vi "RT_Write_DMARS_String.vi"(8 "error in (no error)":errorcluster, 9 "String":string, 11 "FPGA VI Reference Out":refnum<k20>) -> (0 "error out":errorcluster, 3 "FPGA VI Reference Out 2":refnum<k20>)   [LabVIEW 2011]
uses:
  <vilib>/Utility/error.llb/Error Cluster From Error Code.vi
  <vilib>/rvi/errors/niLvFpgaAdjustHostInterfaceError.vi
  <vilib>/RVI Host/nirviSupport.llb/nirviErrorClusterFromErrorCode.vi
  <vilib>/rvi/interface/nirviReadWriteControl/nirviReadWriteControl.xnode
  <vilib>/rvi/interface/nirviMethod/nirviMethod.xnode
  <vilib>/rvi/errors/niLvFpgaMergeErrorWithErrorCode.vi
  <vilib>/FPGAPlugInAG/Dynamic/niLvFpga_WriteFifo_Dynamic.vi
  NiFpgaLv.dll
  <vilib>/rvi/interface/Simulation/niFpgaSimulationCallBeginRW.vi
  <vilib>/rvi/interface/nirviMethod/StockFPGA_InlinedMethodWaitForSingleIRQ.vi
  <vilib>/FPGAPlugInAG/Dynamic/niLvFpga_WaitOnIrq_Dynamic.vi
  <vilib>/FPGAPlugInAG/Dynamic/niLvFpga_AcknowledgeIrq_Dynamic.vi
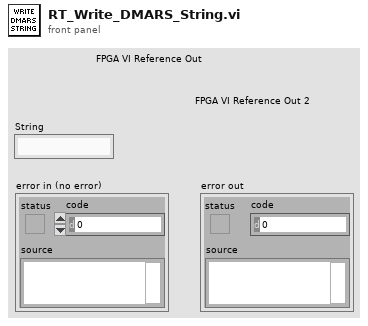
[diagram p1: front panel]
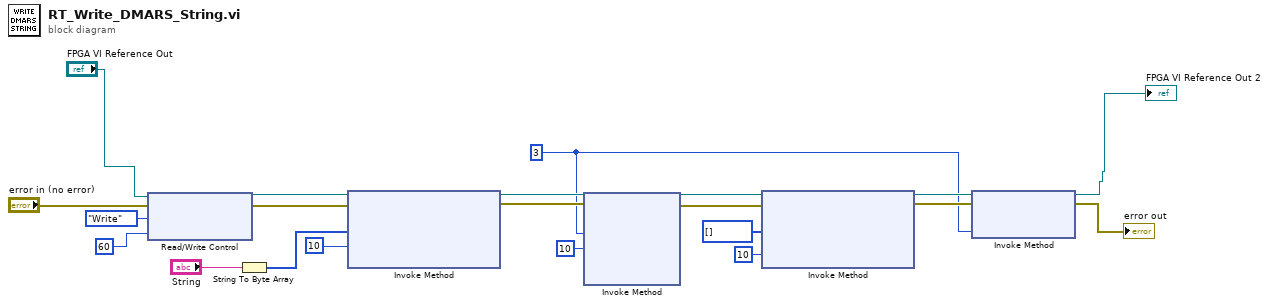
[diagram p0: block diagram]
diagram:
  w6 = 3 ("IRQ Number(s)")
  n1 = xnode "Read/Write Control"("FPGA VI Reference In"="FPGA VI Reference Out", "error in"="error in (no error)", "Op_Write P3"=enum16{"Stand_by", "Write"}."Write" ("Op_Write"), "Bytes-to-Write P3"=60 ("Bytes-to-Read")) -> ("FPGA VI Reference Out"=w10:refnum<k20>, "error out"=w11:errorcluster)
  n2 = String To Byte Array(string="String") -> (unsigned byte array=w20:u8[])
  n3 = xnode "Invoke Method"("FPGA VI Reference In"=w10, "error in"=w11, "Data"=w20, "Timeout (ms)"=10) -> ("FPGA VI Reference Out"=w12:refnum<k20>, "error out"=w13:errorcluster)  [unwired: 1 out]
  n4 = xnode "Invoke Method"("FPGA VI Reference In"=w12, "error in"=w13, "IRQ Number(s)"=w6, "Timeout (ms)"=10) -> ("FPGA VI Reference Out"=w14:refnum<k20>, "error out"=w15:errorcluster)  [unwired: 2 out]
  n5 = xnode "Invoke Method"("FPGA VI Reference In"=w14, "error in"=w15, "Data"=u8[] [], "Timeout (ms)"=10) -> ("FPGA VI Reference Out"=w16:refnum<k20>, "error out"=w17:errorcluster)  [unwired: 1 out]
  n6 = xnode "Invoke Method"("FPGA VI Reference In"=w16, "error in"=w17, "IRQ Number(s)"=w6) -> ("FPGA VI Reference Out"=→"FPGA VI Reference Out 2":refnum<k20>, "error out"=→"error out":errorcluster)
